vi "Create with Type Override.vi"(6 "Type Override":string, 7 "Direction":T1, 8 "error in (no error)":errorcluster, 9 "Custom Config Data":u8[](array[numeric]), 10 "Name":string, 11 "CIFFIFO in":refnum<class "CIF_NIChn_Fifo_U8.lvclass">) -> (0 "error out":errorcluster, 3 "CIFFIFO out":refnum<class "CIF_NIChn_Fifo_U8.lvclass">)   [LabVIEW 2021, in "CIF_NIChn_Fifo_U8.lvclass"]
uses:
  CIF_NIChn_Fifo_U8.lvclass
  D:/dev/Packages/Channel_Manager/src/CIFChannels/CIFChannels.lvclass
  D:/dev/Packages/Channel_Manager/src/CIF_NIChn/NIChn/CIF_NIChn.lvclass
  CIFChannels/Typedef/Direction.ctl
  <vilib>/CIF Foundation/CIF Utilities/Statistics/I64/Stats_I64_CIF_U.lvclass/Stats_I64_CIF_U.ctl
  CIFChannels/Typedef/Disconnect Behavior.ctl
  CIFChannels/CIFChannels.lvclass/CIFChannels.ctl
  CIF_NIChn_Fifo_U8.lvclass/CIF_NIChn_Fifo_U8.ctl
  CIFChannels/Typedef/Channel State.ctl
  NIChn/CIF_NIChn.lvclass/CIF_NIChn.ctl
  c6f1aac1-fdda-4143-8087-f9e7d57e6170.vi
  05c6e502-0377-480c-a15d-085597602460.vi
  CIFChannels/Accessors/Write Channel State.vi
  NIChn/Accessors/Write CIF Channel.vi
  CIFChannels/Accessors/Write Channel Benchmark.vi
  CIFChannels/Accessors/Write Flatten Benchmark.vi
  CIFChannels/Accessors/Write Type.vi
  CIFChannels/SubVIs/Get Type from Class.vi
  ChannelCommon/Utilities/Unflatten FIFO Config.vi
  CIFChannels/Utilities/Apply Flags.vi
  CIFChannels/Accessors/Write Channel Class.vi
  CIFChannels/Accessors/Write Direction.vi
  CIFChannels/Accessors/Write Tag Disconnect Behavior.vi
  CIFChannels/Accessors/Write Name.vi
  CIFChannels/Accessors/Write Custom Config Data.vi
  <vilib>/CIF Foundation/CIF Channels/CIFChannels/SubVIs/Add Error.vi
  c6f1aac1-fdda-4143-8087-f9e7d57e6170.vi/c28b0ead-42ad-4072-80a2-aca7f2bd7ce3.vi
  <vilib>/CIF Foundation/CIF Channels/CIFChannels/SubVIs/CIFServices Fill In Error Info Ex.vi
  <vilib>/CIF Foundation/CIF Channels/CIFChannels/SubVIs/Get dll Path.vi
  c6f1aac1-fdda-4143-8087-f9e7d57e6170.vi/259f1102-a6f3-45ef-83a9-e8a266e5a7b9.vi
  05c6e502-0377-480c-a15d-085597602460.vi/c28b0ead-42ad-4072-80a2-aca7f2bd7ce3.vi
  <vilib>/CIF Foundation/CIF Utilities/DataTypes/Unflatten U64.vi
  ChannelCommon/Utilities/Expand FIFO Flags.vi
  <vilib>/CIF Foundation/CIF Utilities/Errors/Append Error Location.vi
  <vilib>/Utility/LVClass/Get LV Class Name.vi
  <vilib>/CIF Foundation/CIF Utilities/Statistics/I64/Stats_I64_CIF_U.lvclass
  CIFChannels/CIFChannels.lvclass
  ChannelCommon/ChannelCommon.lvlib
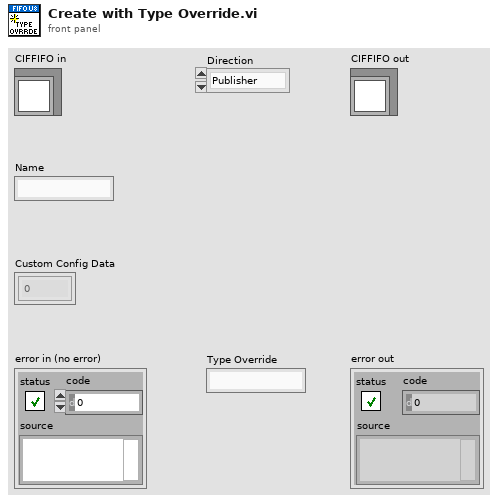
[diagram p1: front panel]
types:
  T1 = typedef "CIFChannels.lvclass/Direction.ctl" = enum16{"Publisher", "Subscriber"}
  T2 = typedef "CIFChannels.lvclass/Disconnect Behavior.ctl" = enum16{"Default value", "Last value", "Error with default"}
  T3 = typedef "CIFChannels.lvclass/Channel State.ctl" = enum16{"Creating", "Disconnected", "Connecting", "Connected", "Destroyed"}
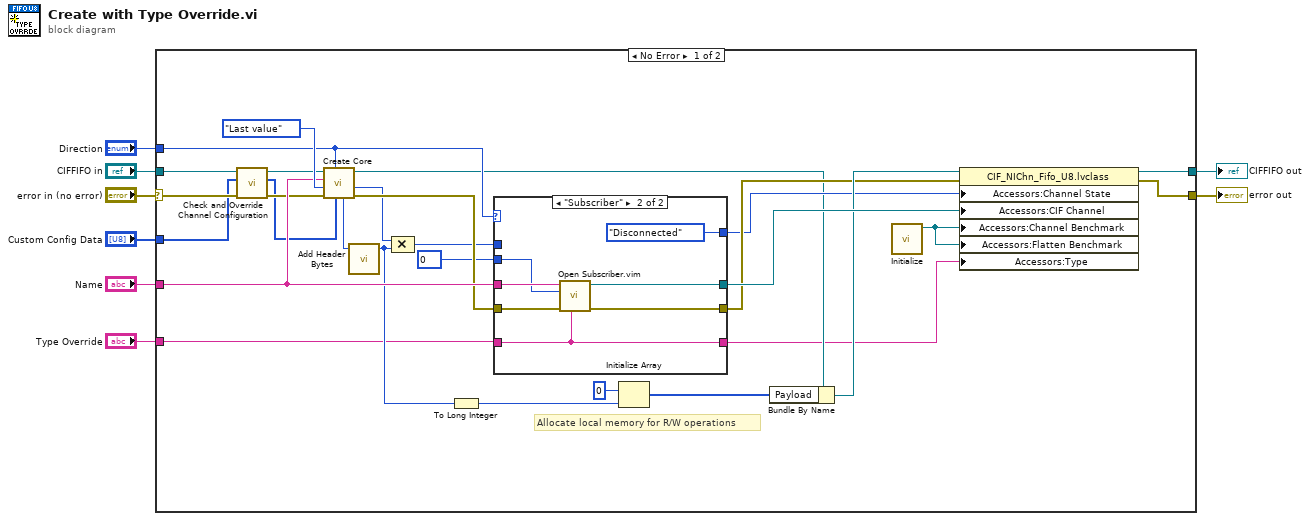
[diagram p0: block diagram]
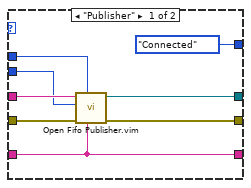
[diagram p2: hidden frame]
diagram:
  n1 = case shown="No Error" "error in (no error)" {
    selector: "error in (no error)" -> [w19 w53]
    tunnel: [w35 w53] -> w7
    tunnel: [w29 w52] -> w5
    tunnel: "CIFFIFO in" -> [w20 w52]
    tunnel: "Name" -> [w34 _]
    tunnel: "Direction" -> [w28 _]
    tunnel: "Custom Config Data" -> [w16 _]
    tunnel: "Type Override" -> [w9 _]
    frame No Error {
      # "Allocate local memory for R/W operations"
      n2 = call-dynamic "Check and Override Channel Configuration.vi"("error in (no error)"=w19, "Custom Config Data in"=w16, "CIFFIFO in"=w20) -> ("error out"=w17:errorcluster, "Custom Config Data out"=w15:u8[], "CIFFIFO out"=w18:refnum<class "CIF_NIChn_Fifo_U8.lvclass">)  [unwired: 6 in]
      n3 = call "Create Core.vi"("Custom Config Data"=w15, "Direction"=w28, "error in (no error)"=w17, "Disconnect Behavior"=Disconnect_Behavior."Last value", "Name"=w34, "CIFChannels in"=w18) -> ("error out"=w33:errorcluster, "Messages"=w13:u64, "CIFChannels out"=w26:refnum<class "CIF_NIChn_Fifo_U8.lvclass">, "Bytes/Msg"=w12:u64)  [unwired: 1 in, 1 out]
      n4 = call "Add Header Bytes.vi"("Bytes/Msg"=w12) -> ("Bytes/Msg with header"=w11:u64)  [unwired: 3 in]
      n5 = Compound Arithmetic op=MULTIPLY(w13, w11) -> (w21:u64)
      n6 = To Long Integer(number=w11) -> (32bit integer=w14:i32)
      n7 = case shown="\"Subscriber\"" w28 {
        tunnel: w34 -> [w44 w50]
        tunnel: w33 -> [w43 w49]
        tunnel: [w40 w46] -> w32
        tunnel: [w41 w47] -> w30
        tunnel: w9 -> [w37 w45]
        tunnel: [Channel_State."Connected" ("Channel State") Channel_State."Disconnected" ("Channel State")] -> w27
        tunnel: u8 0 -> [w39 w48]
        tunnel: w21 -> [w38 _]
        tunnel: [w37 w45] -> w10
        frame "Publisher" {
          n8 = call "Open Fifo Publisher.vim"("Channel Type Description"=w37, "depth"=w38, "error in"=w43, "Input Type"=w39, "Channel Name"=w44) -> ("error out"=w41:errorcluster, "CIF Channel"=w40:refnum<k21>)  [unwired: 5 in]
        }
        frame "Subscriber" {
          n9 = call "Open Subscriber.vim"("Channel Type Description"=w45, "error in"=w49, "Input Type"=w48, "Channel Name"=w50) -> ("error out"=w47:errorcluster, "CIF Channel"=w46:refnum<k21>)  [unwired: 6 in]
        }
      }
      n10 = Initialize Array(u8 0 ("Numeric"), w14) -> (w23:u8[])
      n11 = Bundle By Name(cluster=w26, "Payload"=w23) -> (w31:refnum<class "CIF_NIChn_Fifo_U8.lvclass">)
      n12 = call <vilib>:"Initialize.vi"() -> ("Stats_I64_CIF_U out"=w22:refnum<class "Stats_I64_CIF_U.lvclass">)  [unwired: 10 in, 1 out]
      n13 = property class="CIF_NIChn_Fifo_U8.lvclass"(reference=w31, error in=w30, "Accessors:Channel State"=w27, "Accessors:CIF Channel"=w32, "Accessors:Channel Benchmark"=w22, "Accessors:Flatten Benchmark"=w22, "Accessors:Type"=w10) -> (reference out=w29:refnum<class "CIF_NIChn_Fifo_U8.lvclass">, error out=w35:errorcluster)
    }
    frame Error {
    }
  }
  "error out" <- w7
  "CIFFIFO out" <- w5
